vi "problem_2_part4.vi"() -> ()   [LabVIEW 2020]
panel:
  out "Second Root":dbl format="%#_3g"
  out "First Root":dbl format="%#_3g"
  in  "C":dbl
  in  "B":dbl
  in  "A":dbl
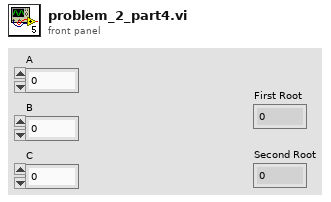
[diagram p1: front panel]
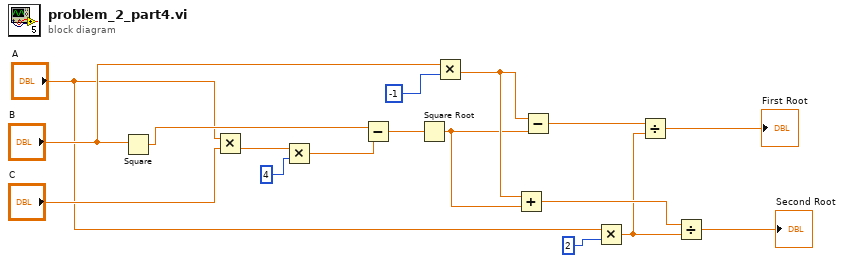
[diagram p0: block diagram]
diagram:
  n1 = Square(x="B") -> (x^2=w14:dbl)
  n2 = Multiply(x="A", y="C") -> (x*y=w16:dbl)
  n3 = Multiply(x=w16, y=4) -> (x*y=w13:dbl)
  n4 = Subtract(x=w14, y=w13) -> (x-y=w12:dbl)
  n5 = Square Root(x=w12) -> (sqrt(x)=w8:dbl)
  n6 = Multiply(x="B", y=-1) -> (x*y=w9:dbl)
  n7 = Add(x=w9, y=w8) -> (x+y=w5:dbl)
  n8 = Subtract(x=w9, y=w8) -> (x-y=w2:dbl)
  n9 = Multiply(x="A", y=2) -> (x*y=w3:dbl)
  n10 = Divide(x=w2, y=w3) -> (x/y=→"First Root":dbl)
  n11 = Divide(x=w5, y=w3) -> (x/y=→"Second Root":dbl)
